vi "myDAQ ASK Communication.vi"() -> ()   [LabVIEW 2009]
uses:
  <vilib>/Analysis/NI_AALBase.lvlib
panel:
  out "Recieved Signal":dbl[](graph)
  out "Recieved Bitstream":bool[](array[boolean])
  out "Received Message":string
  out "Transmit Bitstream":bool[](array[boolean])
  in  "Transmit":bool
  in  "Message  (10 Char)":string="<msg here>"
  in  "stop":bool
  out "Transmit Signal":waveform(dbl)(graph)
  # "ASK Transmitter"
  # "ASK Receiver"
  # "Required connects:  1. Audio Loop Back    (or)  2. Speaker and Microphone"
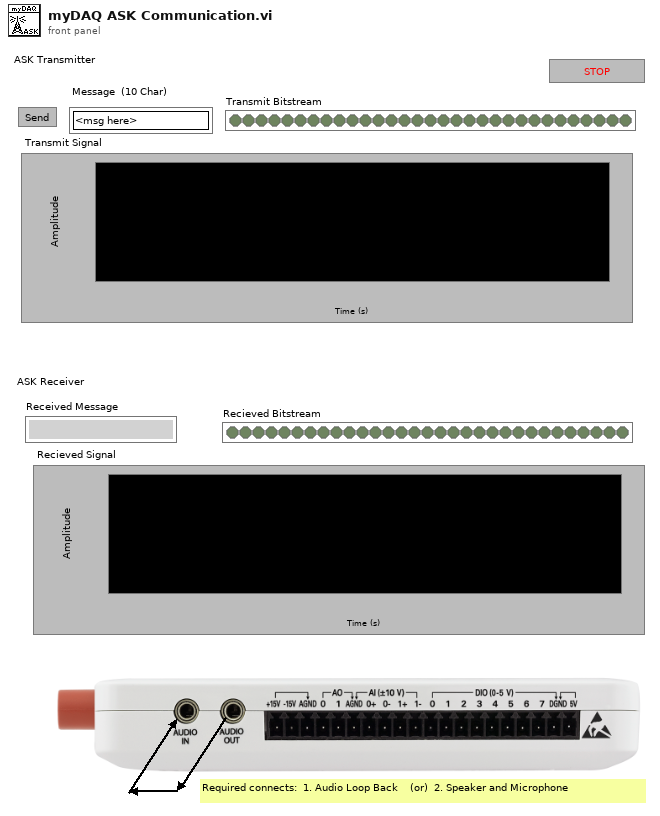
[diagram p1: front panel]
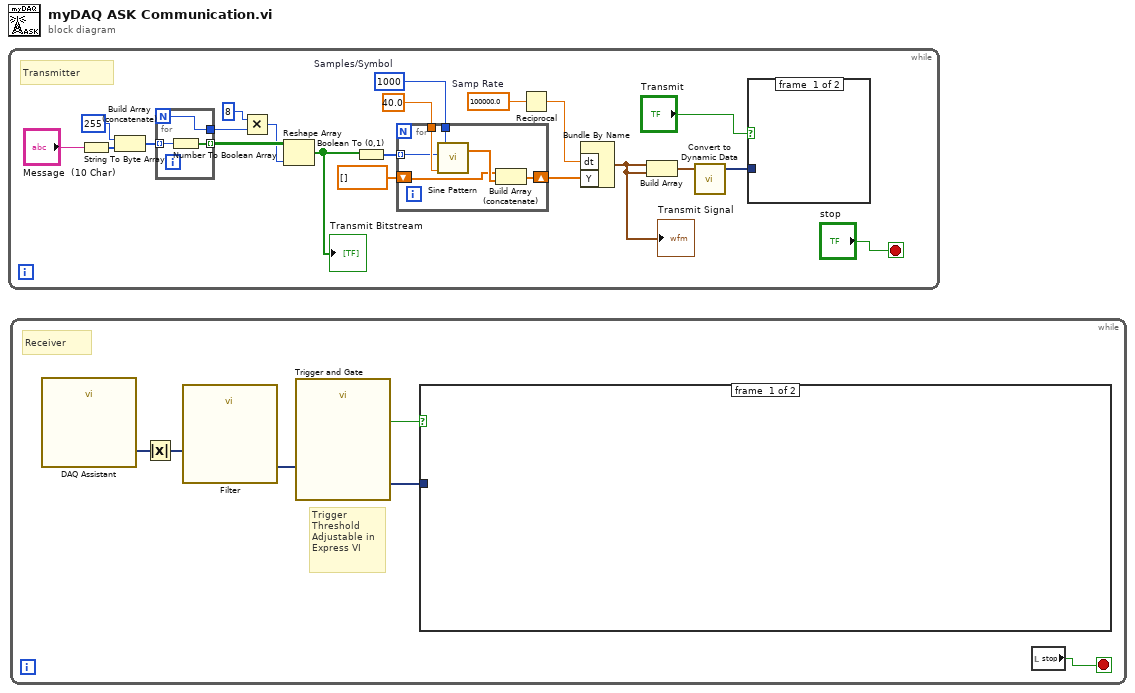
[diagram p0: block diagram]
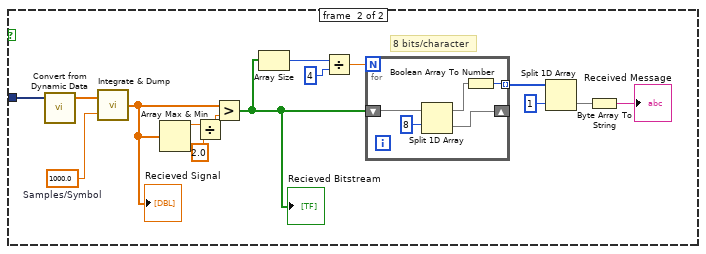
[diagram p2: hidden frame]
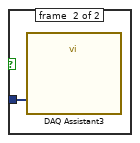
[diagram p3: hidden frame]
diagram:
  n1 = while {
    stop <- "stop" stop-if-true
    w15 = 100000.0  # Samp Rate
    w19 = 1000  # Samples/Symbol
    # "Transmitter"
    n2 = String To Byte Array(string="Message  (10 Char)") -> (unsigned byte array=w10:u8[])
    n3 = Build Array (concatenate)(u8 255, w10) -> (w9:u8[])
    n4 = for {
      N -> [w23]
      tunnel: w9 -> [w25] mode=indexing
      tunnel: [w24] -> w13 mode=indexing
      tunnel: [w23] -> w7
      n5 = Number To Boolean Array(number=w25) -> (Boolean array=w24:bool[])
    }
    n6 = Multiply(x=8 ("y"), y=w7) -> (x*y=w12:i32)
    n7 = Reshape Array(w13, w12) -> (w5:bool[])
    "Transmit Bitstream" <- w5
    n8 = Boolean To (0,1)(Boolean=w5) -> (0, 1=w18:i16[])
    n9 = for {
      shift-right: [w31] -> w14
      shift-left: dbl[] [] -> [w29]
      tunnel: 40.0 ("cycles") -> [w28]
      tunnel: w19 -> [w27]
      tunnel: w18 -> [w26] mode=indexing
      n10 = call <vilib>:"Sine Pattern.vi"("cycles"=w28, "amplitude"=w26, "samples"=w27) -> ("Sinusoidal Pattern"=w30:dbl[])  [unwired: 1 in, 1 out]
      n11 = Build Array (concatenate)(w29, w30) -> (w31:dbl[])
    }
    n12 = Reciprocal(x=w15) -> (1/x=w16:dbl)
    n13 = Bundle By Name("dt"=w16, "Y"=w14) -> (w4:waveform(dbl))  [unwired: 1 in]
    "Transmit Signal" <- w4
    n14 = Build Array(w4, w4) -> (w2:waveform(dbl)[])
    n15 = call "Convert to Dynamic Data"("Array of Waveforms"=w2) -> ("Dynamic Data Type"=w3:dynamicdata)  [unwired: 3 in]
    n16 = case shown="True" "Transmit" {
      tunnel: w3 -> [_ w22]
      frame #0 {
      }
      frame #1 {
        n17 = call "DAQ Assistant3"("data"=w22) -> ()  [unwired: 17 in, 2 out]
      }
    }
  }
  n18 = while {
    stop <- w36 stop-if-true
    # "Receiver"
    # "Trigger Threshold Adjustable in Express VI"
    n19 = call "DAQ Assistant"() -> ("data"=w33:dynamicdata)  [unwired: 16 in, 3 out]
    n20 = Absolute Value(x=w33) -> (abs(x)=w37:dynamicdata)
    n21 = call "Filter"("Signal"=w37) -> ("Filtered Signal"=w32:dynamicdata)  [unwired: 9 in, 1 out]
    n22 = call "Trigger and Gate"("Signals"=w32) -> ("Triggered Signals"=w35:dynamicdata, "Data Available"=w34:bool)  [unwired: 7 in, 2 out]
    n23 = case shown="True" w34 {
      tunnel: w35 -> [_ w42]
      frame #0 {
      }
      frame #1 {
        w51 = 1000.0  # Samples/Symbol
        # "8 bits/character"
        n24 = call "Convert from Dynamic Data"("Dynamic Data Type"=w42) -> ("Array"=w52:dbl[])  [unwired: 3 in]
        n25 = call "Integrate & Dump.vi"("Integration Time (samples)"=w51, "Signal in"=w52) -> ("Signal out"=w39:dbl[])
        "Recieved Signal" <- w39
        n26 = Array Max & Min(array=w39) -> (max value=w41:dbl)  [unwired: 3 out]
        n27 = Divide(x=w41, y=2.0) -> (x/y=w40:dbl)
        n28 = Greater?(x=w39, y=w40) -> (0:w43:bool[])
        "Recieved Bitstream" <- w43
        n29 = Array Size(array=w43) -> (size(s)=w50:i32)
        n30 = Divide(x=w50, y=4) -> (x/y=w48:dbl)
        n31 = for {
          N: w48 -> [_]
          shift-right: [w56] -> _
          shift-left: w43 -> [w57]
          tunnel: [w55] -> w45 mode=indexing
          n32 = Split 1D Array(array=w57, index=8) -> (first subarray=w53:bool[], second subarray=w56:bool[])
          n33 = Boolean Array To Number(Boolean array=w53) -> (number=w55:u32)
        }
        n34 = Split 1D Array(array=w45, index=1) -> (second subarray=w46:u32[])  [unwired: 1 out]
        n35 = Byte Array To String(unsigned byte array=w46) -> (string=→"Received Message":string)
      }
    }
    n36 = local read "stop"() -> (w36:bool)
  }
